vi "MatchRegExJit.vi"(5 "capture index":i32, 7 "Options":cluster{"Compile":u32, "Match":u32, "Jit":u32}={"Compile"=0, "Match"=0, "Jit"=1} {"Jit" format="%.0x"; "Match" format="%.0x"; "Compile" format="%.0x"}, 8 "error in":errorcluster, 9 "offset (0)":i32, 10 "search pattern":string, 11 "string":string) -> (0 "error out":errorcluster, 1 "after substring":string, 2 "match substring":string, 3 "before substring":string, 4 "offset past match":i32, 6 "match offset":i32)   [LabVIEW 2021, in "libpcre2-8.lvlib"]
uses:
  libpcre2-8.lvlib
  Pcre2GetOvectorPointer8.vi
  Pcre2MoOfSubstrNumFmOv.vi
  Pcre2CompileError.vi
  Pcre2FnkCallError.vi
  Pcre2ErrorNull.vi
  Pcre2LibError.vi
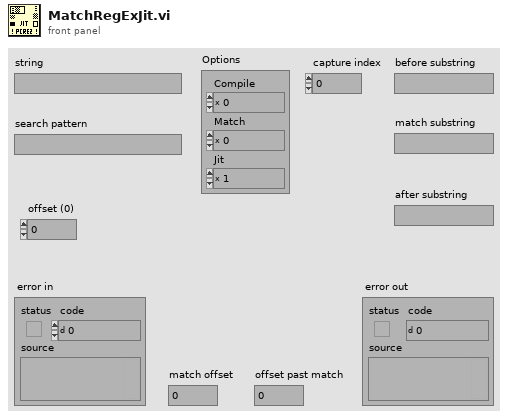
[diagram p1: front panel]
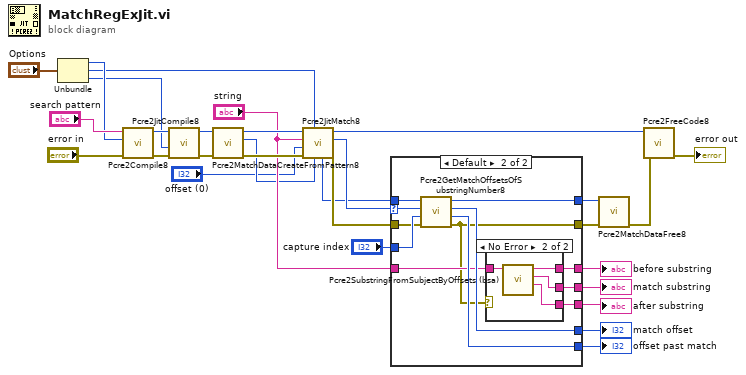
[diagram p0: block diagram]
diagram:
  n1 = Unbundle("Options") -> ("Compile"=w14:u32, "Match"=w13:u32, "Jit"=w2:u32)
  n2 = call "Pcre2Compile8.vi"("error in"="error in", "Options"=w14, "Pattern"="search pattern") -> ("error out"=w5:errorcluster, "pCode"=w6:u64)  [unwired: 7 in]
  n3 = call "Pcre2JitCompile8.vi"("error in"=w5, "Options (1)"=w2, "pCode"=w6) -> ("error out"=w4:errorcluster, "pCode"=w3:u64)  [unwired: 7 in]
  n4 = call "Pcre2MatchDataCreateFromPattern8.vi"("error in"=w4, "pCode"=w3) -> ("error out"=w22:errorcluster, "pMatchData"=w8:u64, "pCode"=w23:u64)  [unwired: 7 in]
  n5 = call "Pcre2JitMatch8.vi"("pMatchData"=w8, "Options"=w13, "error in"=w22, "StartOffset"="offset (0)", "Subject"="string", "pCode"=w23) -> ("error out"=w12:errorcluster, "MatchResult"=w18:i32, "pCode"=w21:u64, "pMatchData"=w9:u64)  [unwired: 2 in]
  n6 = case shown="Default" w18 {
    selector: w18 -> [_ w40]
    tunnel: w9 -> [w33 w45]
    tunnel: [w31 w37] -> w29
    tunnel: [_ w35] -> w28
    tunnel: [_ w36] -> w27
    tunnel: [w33 w44] -> w11
    tunnel: [w30 w43] -> w26
    tunnel: [w30 w42] -> w25
    tunnel: "string" -> [w31 w38]
    tunnel: "capture index" -> [_ w41]
    tunnel: w12 -> [w32 w39]
    tunnel: [w32 w34] -> w10
    frame -1 {
      w30 = -1 ("MatchOffset")
    }
    frame Default {
      n7 = call "Pcre2GetMatchOffsetsOfSubstringNumber8.vi"("error in"=w39, "Number"=w41, "MatchResult"=w40, "pMatchData"=w45) -> ("error out"=w34:errorcluster, "OffsetPastMatch"=w42:i32, "MatchOffset"=w43:i32, "pMatchData"=w44:u64)  [unwired: 4 in]
      n8 = case shown="No Error" w34 {
        tunnel: [w46 w49] -> w37
        tunnel: [_ w47] -> w35
        tunnel: [_ w48] -> w36
        tunnel: w38 -> [w46 w50]
        frame Error {
        }
        frame No Error {
          n9 = call "Pcre2SubstringFromSubjectByOffsets (bsa).vi"("Subject"=w50) -> ("AfterSubstring"=w47:string, "Substring"=w48:string, "BeforeSubstring"=w49:string)  [unwired: 8 in]
        }
      }
    }
  }
  "match offset" <- w26
  "offset past match" <- w25
  "before substring" <- w29
  "match substring" <- w27
  "after substring" <- w28
  n10 = call "Pcre2MatchDataFree8.vi"("error in"=w10, "pMatchData"=w11) -> ("error out"=w20:errorcluster)  [unwired: 9 in]
  n11 = call "Pcre2FreeCode8.vi"("error in"=w20, "pCode"=w21) -> ("error out"=→"error out":errorcluster)  [unwired: 9 in]
